vi "PID_AutoTune_Example.vi"() -> ()   [LabVIEW 2019]
uses:
  <vilib>/Rock Robotics/WPI/ThirdParty/JAS_Junk/TrajLib/TypeDef/PID_CONTROLLER.ctl
  <vilib>/Rock Robotics/WPI/ThirdParty/JAS_Junk/TrajLib/MathUtil_Clamp.vi
  <vilib>/Rock Robotics/WPI/ThirdParty/JAS_Junk/TrajLib/SlewRateLimiter_New.vi
  <vilib>/Rock Robotics/WPI/ThirdParty/JAS_Junk/TrajLib/SlewRateLimiter_Reset.vi
  <vilib>/Rock Robotics/WPI/ThirdParty/JAS_Junk/TrajLib/SlewRateLimiter_Calculate.vi
  <vilib>/Rock Robotics/WPI/ThirdParty/JAS_Junk/TrajLib/SlewRateLimiter_SetRate.vi
  <vilib>/Rock Robotics/WPI/ThirdParty/JAS_Junk/TrajLib/PIDController_AtSetpoint.vi
  <vilib>/Rock Robotics/WPI/ThirdParty/JAS_Junk/TrajLib/PIDController_SetPIDF.vi
  <vilib>/Rock Robotics/WPI/ThirdParty/JAS_Junk/TrajLib/PIDController_SetDerivativeFilter.vi
  <vilib>/Rock Robotics/WPI/ThirdParty/JAS_Junk/TrajLib/PIDController_SetIntegratorRange.vi
  <vilib>/Rock Robotics/WPI/ThirdParty/JAS_Junk/TrajLib/PIDController_SetTolerancePandV.vi
  <vilib>/Rock Robotics/WPI/ThirdParty/JAS_Junk/TrajLib/PIDController_DisableContinousInput.vi
  <vilib>/Rock Robotics/WPI/ThirdParty/JAS_Junk/TrajLib/PIDController_EnableContinousInput.vi
  <vilib>/Rock Robotics/WPI/ThirdParty/JAS_Junk/TrajLib/PIDController_Reset.vi
  <vilib>/Rock Robotics/WPI/ThirdParty/JAS_Junk/TrajLib/PIDController_New.vi
  <vilib>/Rock Robotics/WPI/ThirdParty/JAS_Junk/TrajLib/PIDController_SetOutputLimits.vi
  <vilib>/Rock Robotics/WPI/ThirdParty/JAS_Junk/TrajLib/LinearFilter_ResetToValue.vi
  <vilib>/Rock Robotics/WPI/ThirdParty/JAS_Junk/TrajLib/LinearFilter_Calculate.vi
  <vilib>/Rock Robotics/WPI/ThirdParty/JAS_Junk/TrajLib/PIDController_NewPeriod.vi
  <vilib>/Rock Robotics/SystemInterfaces/NetworkCommunication/NetComm_UsageReport_report.vi
  <vilib>/Rock Robotics/WPI/ThirdParty/JAS_Junk/TrajLib/LinearFilter_MovingAverage.vi
  <vilib>/Rock Robotics/WPI/ThirdParty/JAS_Junk/TrajLib/LinearFilter_LowPassBW1.vi
  <vilib>/Rock Robotics/WPI/ThirdParty/JAS_Junk/TrajLib/LinearFilter_LowPassBW2.vi
  <vilib>/Rock Robotics/WPI/ThirdParty/JAS_Junk/TrajLib/LinearFilter_HighPassBW1.vi
  <vilib>/Rock Robotics/WPI/ThirdParty/JAS_Junk/TrajLib/LinearFilter_HighPassBW2.vi
  <vilib>/Rock Robotics/WPI/ThirdParty/JAS_Junk/TrajLib/Util_LibraryGlobals.vi
  <vilib>/Rock Robotics/WPI/ThirdParty/JAS_Junk/TrajLib/PIDController_AdvCalculate_FF_Sp_Pv.vi
  <vilib>/Rock Robotics/WPI/ThirdParty/JAS_Junk/TrajLib/Trajectory_Library.lvlib
panel:
  out "Plant and Test Data":T1
  out "Tuning Done":bool
  in  "Type of Controller":enum16{"P", "PI", "PID"}(ring)=enum."PI"
  in  "Controller Constant Type":T2(ring)=enum."Ziegler Nicols - Slow"
  in  "Procedure Type":enum16{"Open Loop Step", "Closed Loop Step"}(ring)
  out "New Tuning Parameters":T3
  out "Error Occured":bool
  in  "Tune":bool
  in  "CO Offset":dbl=0.25 format="%#_13g"
  out "Diagnostic Info":T4
  in  "Desired Speed":dbl(slide)=-0.22222222222222499 scale=-10.0..10.0 scale format="%#.1f"
  in  "Tab Control":T5(tab)
  in  "Enable Noise":bool
  in  "Auto / Manual":bool=TRUE
  out "Dash Speed Demand":dbl format="%10.2f"
  out "Dash Speed Target":dbl format="%10.2f"
  out "DashLeft Wheel Speed":dbl(knob)=-2.895988890827539e-05 scale=-15.0..15.0
  out "Left Wheel ErrorFilt":dbl format="%11.3f"
  out "DashLeftMotorOutput":dbl format="%11.3f"
  out "Left Wheel Speed Filt":dbl format="%10.2f"
  out "Duration":dbl format="%11.3f"
  out "Late":dbl format="%11.3f"
  out "SP, PV, CO Left":T6(graph)
  in  "SetPoint Change Rate":dbl=80.0 min=1.0 max=9000.0 format="%14.4f"
  in  "Left Adv PID Limits":T7={"MaxInput"=50.0, "MinInput"=-50.0, "Continuous"=FALSE, "MaxOutput"=1.0, "MinOutput"=-1.0}
  in  "Left PID Error Tolerance":T8={"PositionTolerance"=0.001, "VelocityTolerance"=9.9e+30}
  in  "Left Adv PID Tuning":T9={"Kf"=0.1, "Kp"=0.15, "Ki"=0.1, "Kd"=0.004, "MaximumIntegral"=9.9e+30, "MinimumIntegral"=-9.9e+30, "Filter Derivative"=TRUE}
  out "Left PID Data":T10={"Kp"=0.0, "Ki"=0.0, "Kd"=0.0, "Period"=0.0, "Max_Integral"=0.0, "Min_Integral"=0.0, "Max_Input"=0.0, "Min_Input"=0.0, "Continuous"=FALSE, "PositionError"=0.0, "VelocityError"=0.0, "PrevError"=0.0, "TotalError"=0.0, "PositionTolerance"=0.0, "VelocityTolerance"=0.0, "SetPoint"=0.0, "Kf"=0.0, "Prev_Deriv"=0.0, "Prev_Deriv 2"=0.0, "DerivativeFilter"=FALSE, "Min_Output"=-9.99e+35, "Max_Output"=9.9e+35, "Prev_F_P"=0.0, "Prev_F_P_2"=0.0, "AntiWindupActive"=FALSE, "Measurement"=0.0} {"Measurement" format="%16_6e"; "Prev_F_P_2" format="%16_6e"; "Prev_F_P" format="%16_6e"; "Max_Output" format="%16_6e"; "Min_Output" format="%16_6e"; "Prev_Deriv 2" format="%16_6e"; "Prev_Deriv" format="%16_6e"; "Kf" format="%16_6e"; "SetPoint" format="%16_6e"; "VelocityTolerance" format="%16_6e"; "PositionTolerance" format="%16_6e"; "TotalError" format="%16_6e"; "PrevError" format="%16_6e"; "VelocityError" format="%16_6e"; "PositionError" format="%16_6e"; "Min_Input" format="%16_6e"; "Max_Input" format="%16_6e"; "Min_Integral" format="%16_6e"; "Max_Integral" format="%16_6e"; "Period" format="%16_6e"; "Kd" format="%16_6e"; "Ki" format="%16_6e"; "Kp" format="%16_6e"}
  out "LeftWheelSpeed":dbl
  out "LeftMotorOutput":dbl
  out "SpeedSetpoint":dbl
  in  "SpeedTarget":dbl
  in  "SpeedControlEnabled":bool
  out "LibUsage_Kinematics":i32 format="%20.0f"
  out "LibUsage_TrapezoidProfile":i32 format="%20.0f"
  out "LibUsage_LinearFIlter":i32 format="%20.0f"
  out "LibUsage_Odometry":i32 format="%20.0f"
  out "LibUsage_PIDController":i32 format="%20.0f"
  out "LibUsage_ProfiledPID":i32 format="%20.0f"
  # "PID AutoTune Example"
  # "Enter a desired speed and then press the Set Speed Target \nbutton.  This simulates the joystick input."
  # "FT/SEC"
  # "This value shows the current speed of each wheel.  This is measured by an encoder.  The encoder measures\n speed by counting pulses of the wheel turning and dividing by the time interval.  Total distance change\nis also a result.  This value is called the \"Process Variable\"."
  # "FT/SEC"
  # "FT/SEC"
  # "The Speed Target is rate limited so not to make\nto drastic a change in the desired speed.  (This is\nwhat happens mechanically when pushing the gas\npedal of a real car.)"
  # "This error value shows the error between the current speed\nand the speed demand."
  # "FT/SEC"
  # "This example adds a \"Manual\" mode so that the still operates\nif the encoder fails."
  # "FT/SEC"
  # "This value shows the current motor output demand.  This could also be a motor speed demand and \nanother closed loop controller would control the motor speed.  In this simple example this value is \nused to drive the simulated motor directly.  This motor demand is called the \"Control Output\"."
  # "Enables some simulated process noise"
  # "FT/SEC/SEC"
  # "These are the tuning parameters for the PID VI"
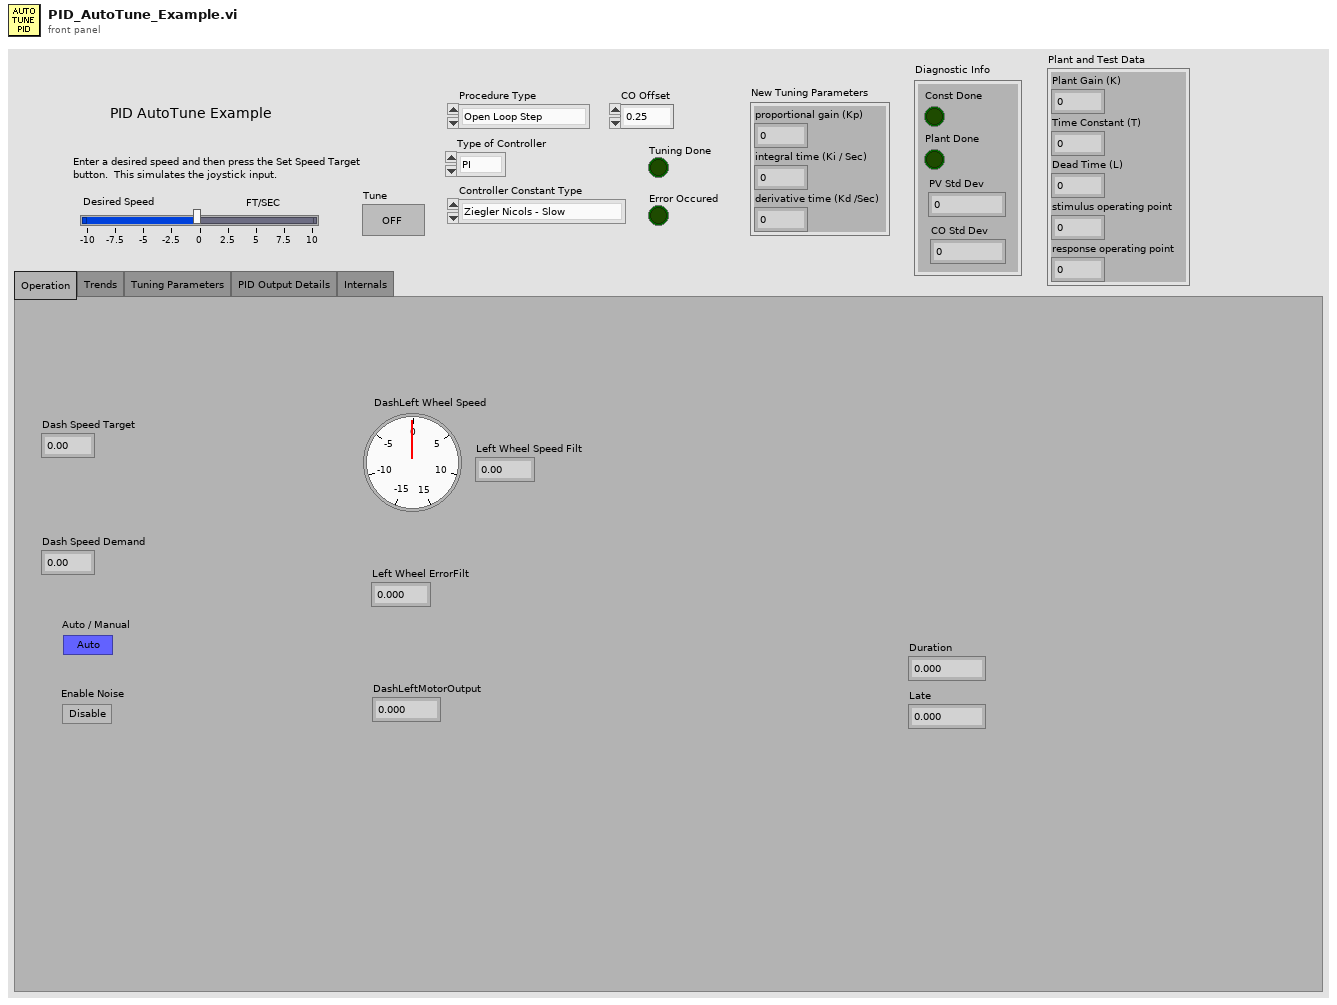
[diagram p1: front panel]
types:
  T1 = cluster{"Plant Gain (K)":dbl, "Time Constant (T)":dbl, "Dead Time (L)":dbl, "stimulus operating point":dbl, "response operating point":dbl}
  T2 = enum16{"Ziegler Nicols - Fast", "Ziegler Nicols - Normal", "Ziegler Nicols - Slow", "CHR regulator - 0% overshoot", "CHR regulator - 20% overshoot", "CHR servo - 0 % overshoot", "CHR servo - 20% overshoot"}
  T3 = cluster{"proportional gain (Kp)":dbl, "integral time (Ki / Sec)":dbl, "derivative time (Kd /Sec)":dbl}
  T4 = cluster{"Const Done":bool, "Plant Done":bool, "PV Std Dev":dbl, "CO Std Dev":dbl}
  T5 = enum32{"Operation", "Trends", "Tuning Parameters", "PID Output Details", "Internals"}
  T6 = cluster{"MotorDemand":dbl, "CurrentSetpoint":dbl, "CurrentPosition":dbl}
  T7 = cluster{"MaxInput":dbl, "MinInput":dbl, "Continuous":bool, "MaxOutput":dbl, "MinOutput":dbl}
  T8 = cluster{"PositionTolerance":dbl, "VelocityTolerance":dbl}
  T9 = cluster{"Kf":dbl, "Kp":dbl, "Ki":dbl, "Kd":dbl, "MaximumIntegral":dbl, "MinimumIntegral":dbl, "Filter Derivative":bool}
  T10 = typedef "Trajectory_Library.lvlib/PID_CONTROLLER.ctl" = cluster{"Kp":dbl, "Ki":dbl, "Kd":dbl, "Period":dbl, "Max_Integral":dbl, "Min_Integral":dbl, "Max_Input":dbl, "Min_Input":dbl, "Continuous":bool, "PositionError":dbl, "VelocityError":dbl, "PrevError":dbl, "TotalError":dbl, "PositionTolerance":dbl, "VelocityTolerance":dbl, "SetPoint":dbl, "Kf":dbl, "Prev_Deriv":dbl, "Prev_Deriv 2":dbl, "DerivativeFilter":bool, "Min_Output":dbl, "Max_Output":dbl, "Prev_F_P":dbl, "Prev_F_P_2":dbl, "AntiWindupActive":bool, "Measurement":dbl}
  T11 = enum16{"Moving Average", "Low Pass 1st Order Butterworth", "Low Pass 2nd Order Butterworth", "High Pass 1st Order Butterworth", "High Pass 2nd Order Butterworth"}
  T12 = cluster{"LeftMotorOutput":dbl, "SpeedSetpoint":dbl, "LeftWheelSpeed":dbl}
  T13 = cluster{"Controller Constant Type":enum16{"Ziegler Nicols - Fast", "Ziegler Nicols - Normal", "Ziegler Nicols - Slow", "CHR regulator - 0% overshoot", "CHR regulator - 20% overshoot", "CHR servo - 0 % overshoot", "CHR servo - 20% overshoot"}, "Type of Controller":enum16{"P", "PI", "PID"}, "CO Offset":dbl, "Kn":dbl, "Tuning Tolerance":dbl, "Plant Tolerance":dbl, "Newest Avg Time ":i32, "Long Ave Time":i32}
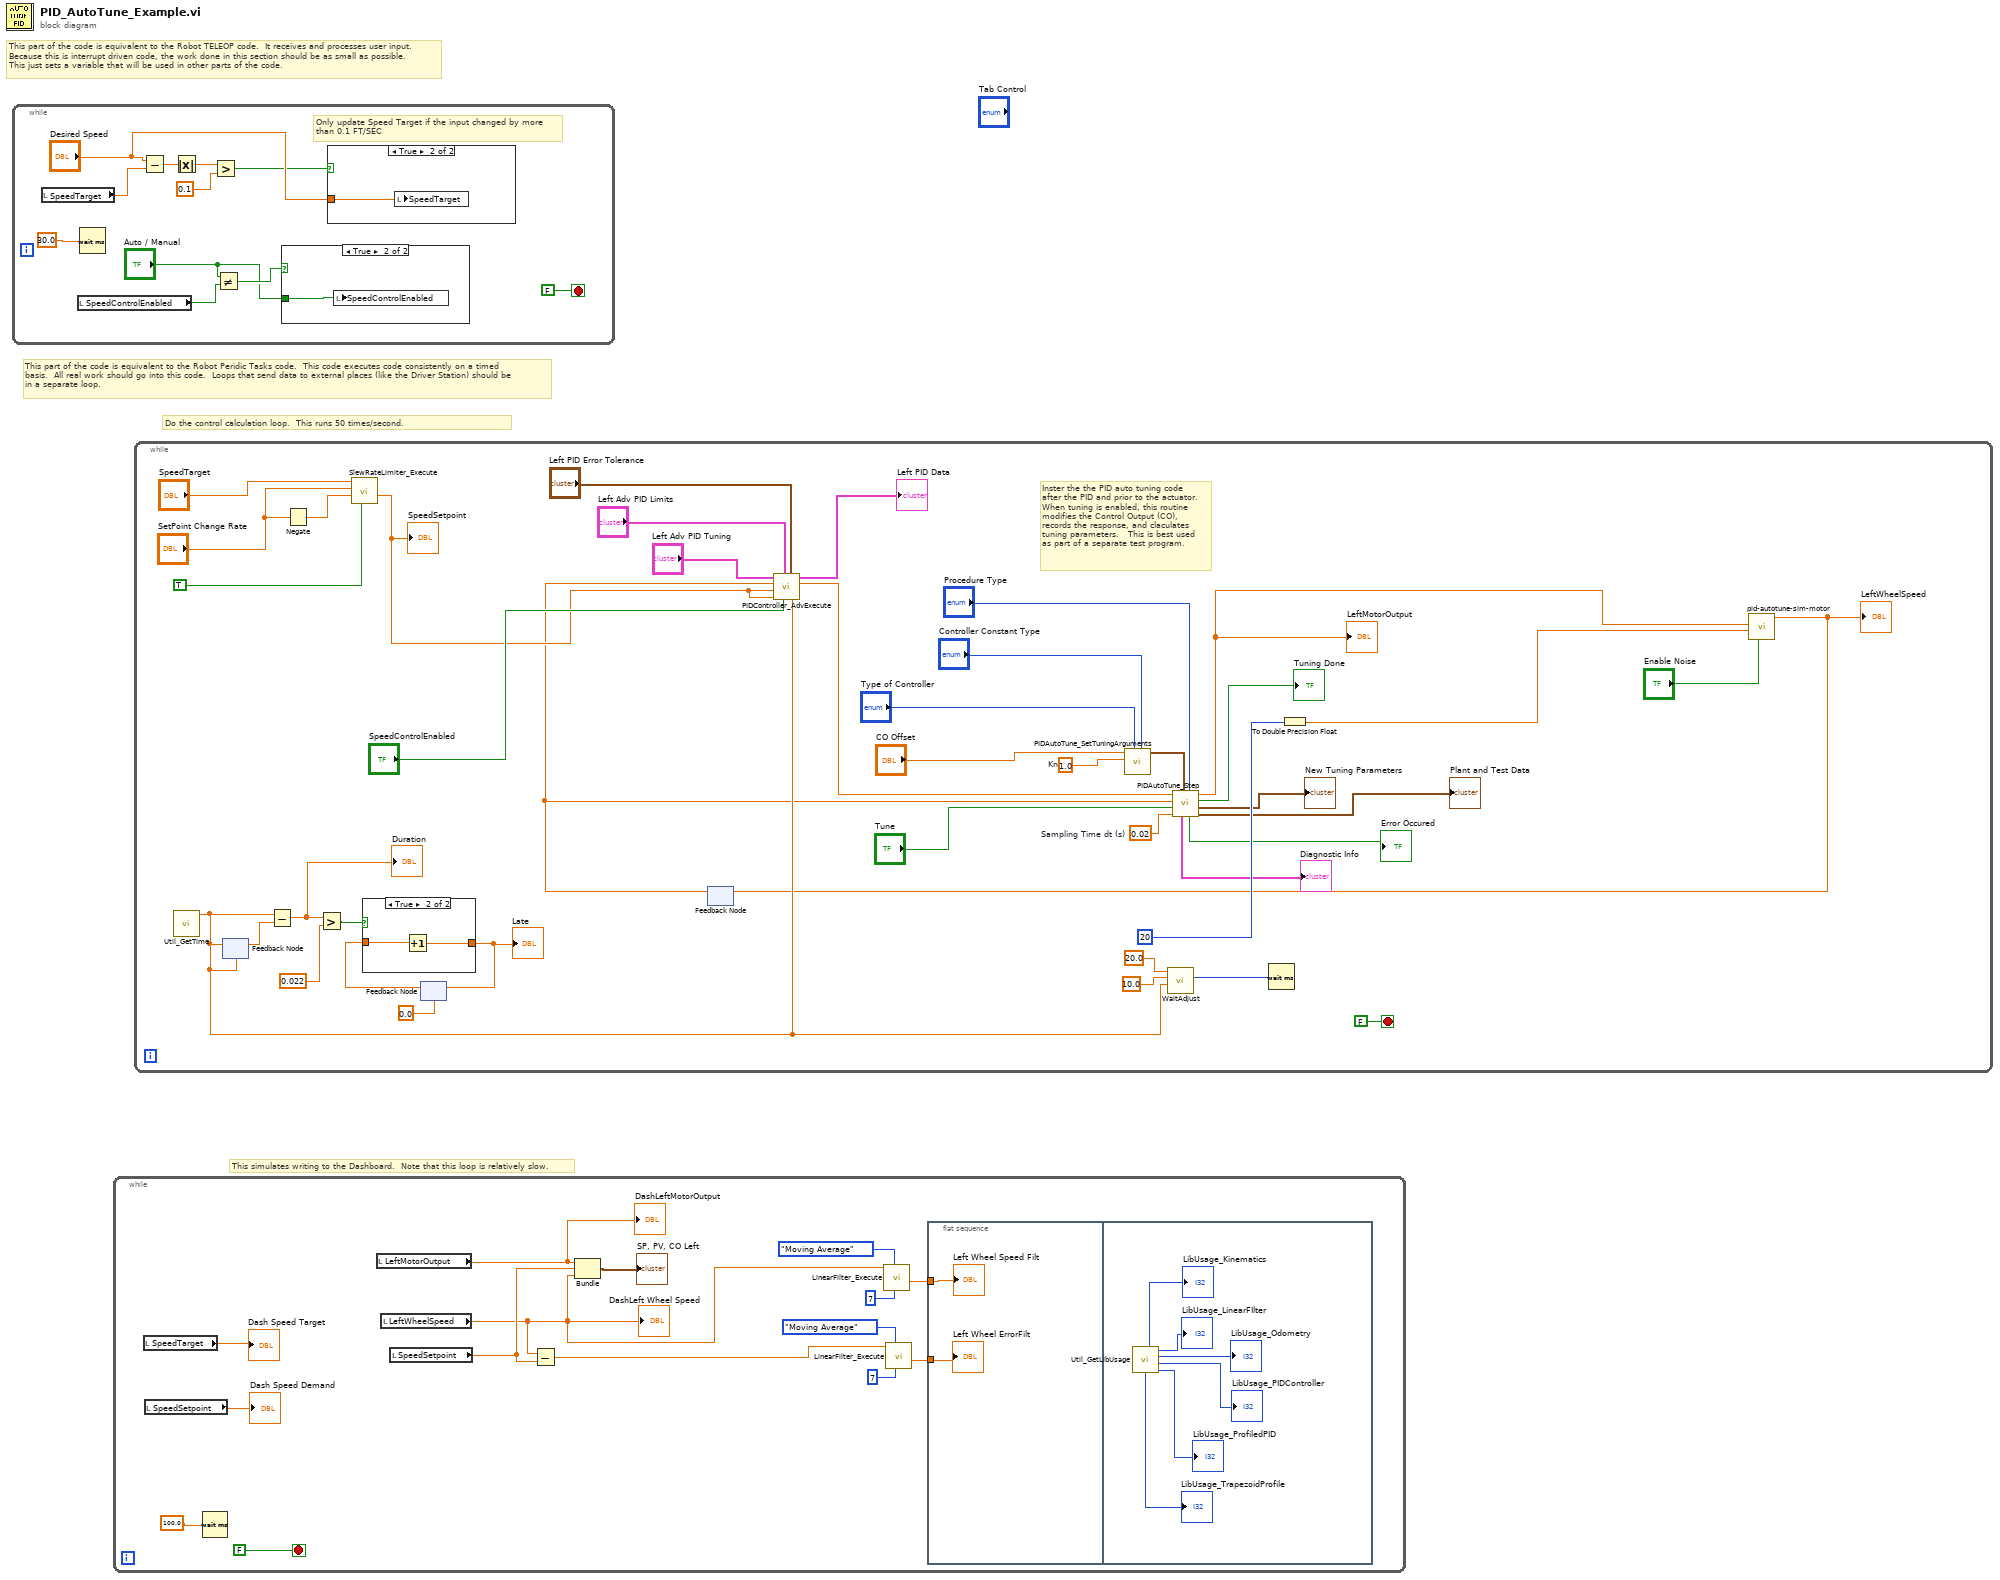
[diagram p0: block diagram]
diagram:
  # "This simulates writing to the Dashboard.  Note that this loop is relatively slow."
  # "Do the control calculation loop.  This runs 50 times/second."
  # "This part of the code is equivalent to the Robot Peridic Tasks code.  This code executes code consistently on a timed\nbasis.  All real work should go into this code.  Loops that send data to external places (like the Driver Station) should be \nin a separate loop."
  # "This part of the code is equivalent to the Robot TELEOP code.  It receives and processes user input.\nBecause this is interrupt driven code, the work done in this section should be as small as possible.\nThis just sets a variable that will be used in other parts of the code."
  n1 = while {
    stop <- FALSE stop-if-true
    # "Only update Speed Target if the input changed by more\nthan 0.1 FT/SEC"
    n2 = local read "SpeedTarget"() -> (w10:dbl)
    n3 = local read "SpeedControlEnabled"() -> (w2:bool)
    n4 = Wait (ms)(milliseconds to wait=30.0) -> ()  [unwired: 1 out]
    n5 = Subtract(x="Desired Speed", y=w10) -> (x-y=w9:dbl)
    n6 = Absolute Value(x=w9) -> (abs(x)=w8:dbl)
    n7 = Greater?(x=w8, y=0.1) -> (0:w5:bool)
    n8 = Not Equal?(x="Auto / Manual", y=w2) -> (x != y?=w3:bool)
    n9 = case shown="True" w3 {
      tunnel: "Auto / Manual" -> [_ w12]
      frame False {
      }
      frame True {
        n10 = local write "SpeedControlEnabled"(w12) -> ()
      }
    }
    n11 = case shown="True" w5 {
      tunnel: "Desired Speed" -> [_ w13]
      frame False {
      }
      frame True {
        n12 = local write "SpeedTarget"(w13) -> ()
      }
    }
  }
  n13 = while {
    stop <- FALSE stop-if-true
    n14 = local read "SpeedTarget"() -> (→"Dash Speed Target":dbl)
    n15 = local read "SpeedSetpoint"() -> (→"Dash Speed Demand":dbl)
    n16 = Wait (ms)(milliseconds to wait=100.0) -> ()  [unwired: 1 out]
    n17 = local read "LeftMotorOutput"() -> (w23:dbl)
    "DashLeftMotorOutput" <- w23
    n18 = local read "LeftWheelSpeed"() -> (w19:dbl)
    "DashLeft Wheel Speed" <- w19
    n19 = local read "SpeedSetpoint"() -> (w22:dbl)
    n20 = Subtract(x=w19, y=w22) -> (x-y=w15:dbl)
    n21 = Bundle("LeftMotorOutput"=w23, "SpeedSetpoint"=w22, "LeftWheelSpeed"=w19) -> (→"SP, PV, CO Left":T12)  [unwired: 1 in]
    n22 = call <vilib>:"LinearFilter_Execute.vi"("Samples"=7, "Filter Type"=T11."Moving Average", "Input"=w19) -> ("Output"=w18:dbl)  [unwired: 7 in, 1 out]
    n23 = call <vilib>:"LinearFilter_Execute.vi"("Samples"=7, "Filter Type"=T11."Moving Average", "Input"=w15) -> ("Output"=w14:dbl)  [unwired: 7 in, 1 out]
    n24 = flat-sequence {
      tunnel: w18 -> [w30]
      tunnel: w14 -> [w29]
      frame #0 {
        "Left Wheel ErrorFilt" <- w29
        "Left Wheel Speed Filt" <- w30
      }
      frame #1 {
        n25 = call <vilib>:"Util_GetLibUsage.vi"() -> ("LibUsage_ProfiledPID"=→"LibUsage_ProfiledPID":i32, "LibUsage_PIDController"=→"LibUsage_PIDController":i32, "LibUsage_Odometry"=→"LibUsage_Odometry":i32, "LibUsage_LinearFIlter"=→"LibUsage_LinearFIlter":i32, "LibUsage_TrapezoidProfile"=→"LibUsage_TrapezoidProfile":i32, "LibUsage_Kinematics"=→"LibUsage_Kinematics":i32)  [unwired: 6 in]
      }
    }
  }
  n26 = while {
    stop <- FALSE stop-if-true
    w59 = 0.02  # Sampling Time dt (s)
    w58 = 1.0  # Kn
    # "Inster the the PID auto tuning code\nafter the PID and prior to the actuator.\nWhen tuning is enabled, this routine\nmodifies the Control Output (CO), \nrecords the response, and claculates\ntuning parameters.   This is best used\nas part of a separate test program."
    n27 = call <vilib>:"Util_GetTime.vi"() -> ("FPGA_Time_Seconds"=w60:dbl)  [unwired: 10 in, 1 out]
    n28 = feedback #1(w60) -> (w74:dbl)
    n29 = feedback-in #1(w60) -> ()
    n30 = Subtract(x=w60, y=w74) -> (x-y=w72:dbl)
    "Duration" <- w72
    n31 = Negate(x="SetPoint Change Rate") -> (-x=w41:dbl)
    n32 = Greater?(x=w72, y=0.022) -> (0:w73:bool)
    n33 = call <vilib>:"SlewRateLimiter_Execute.vi"("Enable"=TRUE, "NegativeRate"=w41, "PositiveRate"="SetPoint Change Rate", "Input"="SpeedTarget") -> ("Output"=w66:dbl)  [unwired: 6 in, 1 out]
    "SpeedSetpoint" <- w66
    n34 = feedback #2(0.0) -> (w75:dbl)
    n35 = case shown="True" w73 {
      tunnel: [w79 w81] -> w76
      tunnel: w75 -> [w79 w80]
      frame False {
      }
      frame True {
        n36 = Increment(x=w80) -> (x+1=w81:dbl)
      }
    }
    "Late" <- w76
    n37 = feedback-in #2(w76) -> ()
    n38 = feedback #3() -> (w51:dbl)  [unwired: 1 in]
    n39 = call <vilib>:"PIDController_AdvExecute.vi"("Time"=w60, "PID Error Tolerance"="Left PID Error Tolerance", "Auto"="SpeedControlEnabled", "Adv PID Limits"="Left Adv PID Limits", "FF-FeedForward"=w66, "SP-SetPoint"=w66, "PV-Measurement"=w51, "Adv PID Tuning"="Left Adv PID Tuning") -> ("CO-ControlOutput"=w52:dbl, "out PID_CONTROLLER"=→"Left PID Data":T10)  [unwired: 1 in, 1 out]
    n40 = call <vilib>:"PIDAutoTune_SetTuningArguments.vi"("Controller Constant Type"="Controller Constant Type", "Type of Controller"="Type of Controller", "Kn"=w58, "CO Offset"="CO Offset") -> ("Configuration Parameters"=w53:T13)  [unwired: 7 in]
    n41 = call <vilib>:"WaitAdjust.vi"("Time_SEC"=w60, "MaxDeviation_MS"=10.0, "DesiredLoopTime_MS"=20.0) -> ("AdjustedWaitTime_MS"=w61:u32)  [unwired: 7 in, 1 out]
    n42 = call <vilib>:"PIDAutoTune_Step.vi"("Procedure Type"="Procedure Type", "Configuration Parameters"=w53, "Sampling Time dt (s)"=w59, "Tune"="Tune", "Measurement  (PV)"=w51, "Control Output (Co)"=w52) -> ("Plant and Test Data"=→"Plant and Test Data":T1, "New Tuning Parameters"=→"New Tuning Parameters":T3, "Tuning Done"=→"Tuning Done":bool, "Adj CO"=w39:dbl, "Error Occured"=→"Error Occured":bool, "Diagnostic Info"=→"Diagnostic Info":T4)
    "LeftMotorOutput" <- w39
    n43 = Wait (ms)(milliseconds to wait=w61) -> ()  [unwired: 1 out]
    n44 = To Double Precision Float(number=u32 20 ("milliseconds to wait")) -> (double precision float=w38:dbl)
    n45 = call "pid-autotune-sim-motor.vi"("Use Noise"="Enable Noise", "Cycle Time"=w38, "CO-ControlOutput"=w39) -> ("Motor Speed"=w40:dbl)  [unwired: 8 in]
    "LeftWheelSpeed" <- w40
    n46 = feedback-in #3(w40) -> ()
  }
